vi "Compute Plots Convolution Product v2.vi"(6 "Step":dbl, 8 "Error In":errorcluster, 9 "Period":dbl, 10 "Plot 2 (kernel)":T1, 11 "Plot 1 (function)":T1) -> (0 "Error Out":errorcluster, 1 "CPU (s)":dbl, 3 "Convolution Product":T1)   [LabVIEW 2021, in "Fits.lvlib"]
uses:
  Fits.lvlib
  Graphs/XY Graph/XY Graph Plot Data.ctl
  a860c85f-9c4a-482a-b616-24d241287ae4.vi
  Graphs/XY Graph/XY Graph Add-Ons.lvlib
  Time/Time.lvlib
  Utilities/Utilities.lvlib
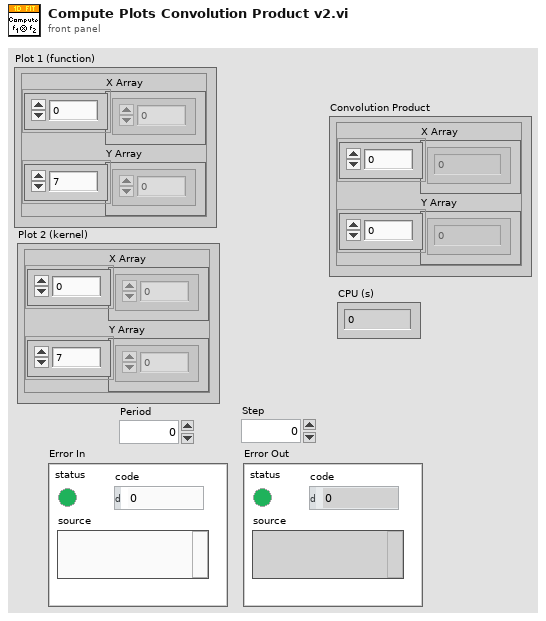
[diagram p1: front panel]
types:
  T1 = typedef "XY Graph Add-Ons.lvlib/XY Graph Plot Data.ctl" = cluster{"X Array":dbl[], "Y Array":dbl[]}
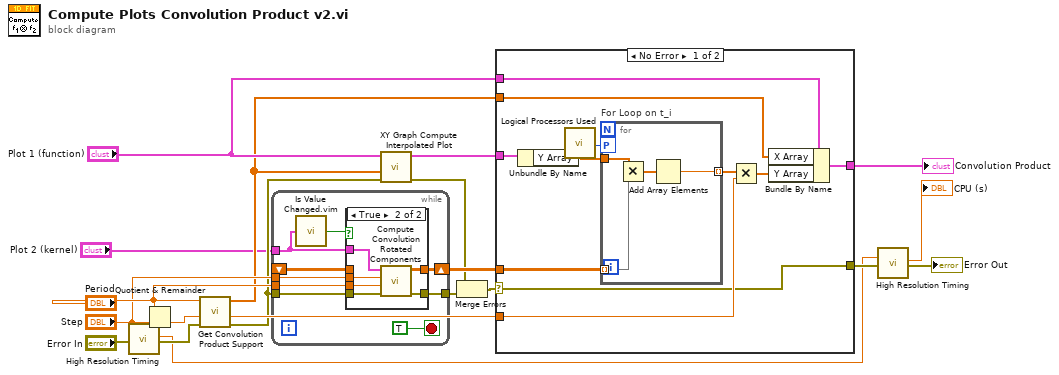
[diagram p0: block diagram]
diagram:
  n1 = call "High Resolution Timing.vi"("Error In"="Error In") -> ("elapsed (relative) seconds"=w3:dbl, "Error Out"=w5:errorcluster)  [unwired: 16 in, 1 out]
  n2 = Quotient & Remainder(x="Period", y="Step") -> (floor(x/y)=w20:dbl)  [unwired: 1 out]
  n3 = call "Get Convolution Product Support.vi"("Error In"=w5, "# Values"=w20, "IRF Period"="Period") -> ("Error Out"=w10:errorcluster, "Step"=w18:dbl, "Ramp"=w13:dbl[])  [unwired: 6 in]
  n4 = while {
    tunnel: "Period" -> [w29]
    tunnel: "Step" -> [w28]
    tunnel: "Plot 2 (kernel)" -> [w24]
    tunnel: w10 -> [w26]
    tunnel: [w25] -> w8
    shift-right: [w27] -> w11
    shift-left: _ -> [w22]
    stop <- TRUE stop-if-true
    n5 = call "Is Value Changed.vim"("value"=w24) -> ("changed or first call?"=w23:bool)
    n6 = case shown="True" w23 {
      tunnel: w29 -> [_ w37]
      tunnel: w28 -> [_ w36]
      tunnel: [w30 w35] -> w27
      tunnel: w26 -> [w31 w34]
      tunnel: [w31 w33] -> w25
      tunnel: w24 -> [_ w32]
      tunnel: w22 -> [w30 _]
      frame False {
      }
      frame True {
        n7 = call "Compute Convolution Rotated Components.vi"("Error In"=w34, "Period"=w37, "Step"=w36, "Plot"=w32) -> ("Error Out"=w33:errorcluster, "Convolution Kernels"=w35:dbl[][])  [unwired: 6 in]
      }
    }
  }
  n8 = call "XY Graph Compute Interpolated Plot.vi"("Error In"=w10, "Ramp"=w13, "Plot"="Plot 1 (function)") -> ("Error Out"=w9:errorcluster, "Interpolated Plot"=w12:T1)  [unwired: 7 in]
  n9 = Merge Errors(w9, w8) -> (w7:errorcluster)
  n10 = case shown="No Error" w7 {
    selector: w7 -> [w39 w54]
    tunnel: w18 -> [w48 _]
    tunnel: [w45 w53] -> w17
    tunnel: "Plot 1 (function)" -> [w44 w53]
    tunnel: w13 -> [w43 _]
    tunnel: w12 -> [w42 _]
    tunnel: w11 -> [w40 _]
    tunnel: [w39 w54] -> w6
    frame No Error {
      n11 = Unbundle By Name(w42) -> ("Y Array"=w41:dbl[])
      n12 = call "Logical Processors Used.vi"() -> ("# Logical Processor Used"=w38:i32)  [unwired: 6 in]
      n13 = for "For Loop on t_i" {
        tunnel: w41 -> [w52]
        tunnel: [w50] -> w47 mode=indexing
        tunnel: w40 -> [w49] mode=indexing
        workers-P: w38 -> [_]
        n14 = Multiply(x=w52, y=w49) -> (x*y=w51:dbl[])
        n15 = Add Array Elements(numeric array=w51) -> (sum=w50:dbl)
      }
      n16 = Multiply(x=w47, y=w48) -> (x*y=w46:dbl[])
      n17 = Bundle By Name(cluster=w44, "X Array"=w43, "Y Array"=w46) -> (w45:T1)
    }
    frame Error {
    }
  }
  "Convolution Product" <- w17
  n18 = call "High Resolution Timing.vi"("relative seconds (NaN)"=w3, "Error In"=w6) -> ("elapsed (relative) seconds"=→"CPU (s)":dbl, "Error Out"=→"Error Out":errorcluster)  [unwired: 15 in, 1 out]
